vi "detect_circle_gray_subVI.vi"(8 "error in (no error)":errorcluster, 11 "Image Out 2":T1(plugin-control)) -> (0 "error out":errorcluster, 2 "Circles (Shape Detection 1)":T2(array[cluster]) {"Position"."Y" format="%.2f"; "Position"."X" format="%.2f"}, 3 "Image Out":T1(plugin-control))   [LabVIEW 2020]
uses:
  <vilib>/vision/NI_Vision_Development_Module.lvlib
panel:
  out "Number of Matches Returned":i32
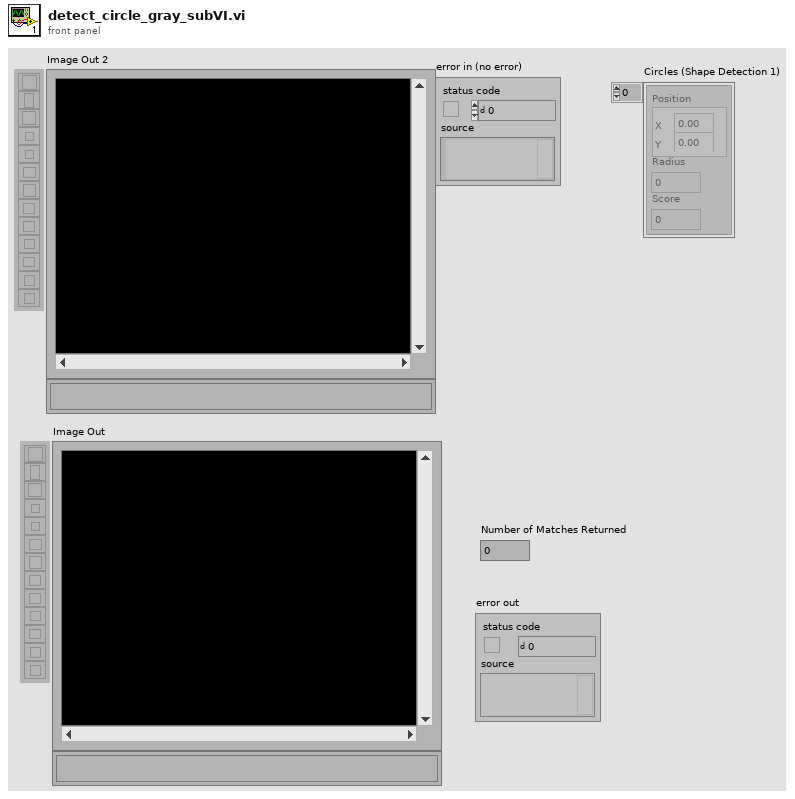
[diagram p1: front panel]
types:
  T1 = typedef "IMAQ Image.ctl" = refnum<image>
  T2 = cluster{"Position":cluster{"X":sgl, "Y":sgl}, "Radius":dbl, "Score":dbl}[]
  T3 = typedef "Image Type" = u32
  T4 = typedef "IMAQ Circle" = cluster{"Center X":i32, "Center Y":i32, "Inner Radius":i32, "Outer Radius":i32, "Start Angle":dbl, "End Angle":dbl}
  T5 = typedef "ROI Descriptor" = cluster{"Global Rectangle":i32[], "Contours":cluster{"ID":enum32{"External", "Internal"}, "Type":u32, "Coordinates":i32[]}[]}
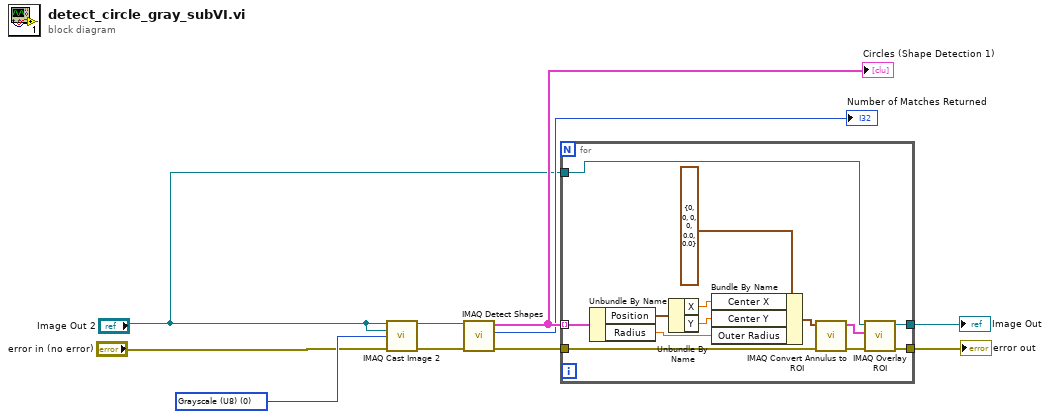
[diagram p0: block diagram]
diagram:
  w3 = T3 0 items=["Grayscale (U8)", "Grayscale (I16)", "Grayscale (SGL)", "Complex (CSG)", "RGB (U32)", "HSL (U32)", "RGB (U64)", "Grayscale (U16)"] ("Image Type")
  n1 = call "IMAQ Cast Image 2"("Image Src"="Image Out 2", "Image Dst"="Image Out 2", "Image Type"=w3, "error in (no error)"="error in (no error)") -> ("Image Dst Out"=w4:T1, "error out"=w5:errorcluster)  [unwired: 10 in]
  n2 = call-poly "IMAQ Detect Shapes"("error in (no error)"=w5, "Image"=w4) -> ("error out"=w7:errorcluster, "Number of Matches Returned"=→"Number of Matches Returned":i32, "Circles"=w10:T2)  [unwired: 5 in, 2 out]
  "Circles (Shape Detection 1)" <- w10
  n3 = for {
    tunnel: w10 -> [w17] mode=indexing
    tunnel: "Image Out 2" -> [w16]
    tunnel: [w15] -> w9
    tunnel: w7 -> [w13]
    tunnel: [w11] -> w6
    n4 = Unbundle By Name(w17) -> ("Position"=w21:cluster{"X":sgl, "Y":sgl}, "Radius"=w18:dbl)
    n5 = Unbundle By Name(w21) -> ("X"=w20:sgl, "Y"=w19:sgl)
    n6 = Bundle By Name(cluster=T4 {"Center X"=0, "Center Y"=0, "Inner Radius"=0, "Outer Radius"=0, "Start Angle"=0.0, "End Angle"=0.0} ("Annulus"), "Center X"=w20, "Center Y"=w19, "Outer Radius"=w18) -> (w23:T4)
    n7 = call "IMAQ Convert Annulus to ROI"("error in (no error)"=w13, "Annulus"=w23) -> ("error out"=w12:errorcluster, "ROI Descriptor"=w14:T5)  [unwired: 7 in]
    n8 = call "IMAQ Overlay ROI"("error in (no error)"=w12, "ROI Descriptor"=w14, "Image"=w16) -> ("error out"=w11:errorcluster, "Image Out"=w15:T1)  [unwired: 7 in]
  }
  "error out" <- w6
  "Image Out" <- w9
